vi "Primary Velocity.vi"(0 "Primary Average Density":dbl, 1 "Pipe X-SectionArea":dbl, 5 "Primary Hot Density":dbl, 7 "Primary Cold Density":dbl, 9 "Pri Mass Flow":dbl, 12 "RX X-Section":dbl, 13 "Numeric":dbl) -> (2 "Cold Leg Velocity (m/s)":dbl, 3 "Hot Leg Velocity (m/s)":dbl, 4 "MHX Velocity (m/s)":dbl, 6 "Velocity (m/s) 2":dbl, 8 "Velocity (m/s) 4":dbl, 10 "Velocity (m/s) 3":dbl, 14 "RX Velocity (m/s)":dbl, 15 "Velocity (m/s)":dbl)   [LabVIEW 2019]
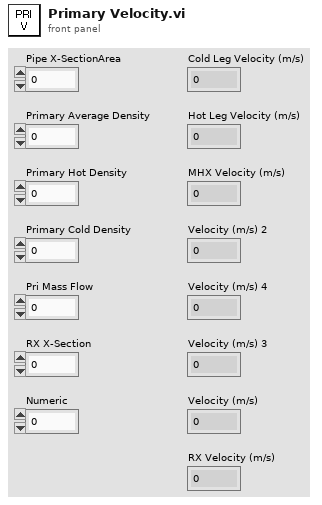
[diagram p1: front panel]
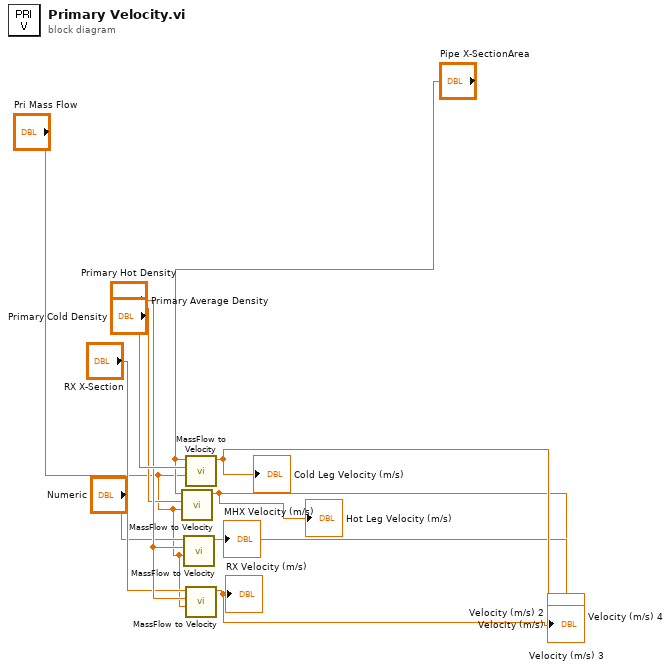
[diagram p0: block diagram]
diagram:
  n1 = call "MassFlow to Velocity.vi"("Mass Flow (kg/s)"="Pri Mass Flow", "Density (kg/m^3)"="Primary Hot Density", "Area (m^2)"="Pipe X-SectionArea") -> ("Velocity (m/s)"=→"Hot Leg Velocity (m/s)" →"Velocity (m/s) 4":dbl)  [unwired: 8 in]
  n2 = call "MassFlow to Velocity.vi"("Mass Flow (kg/s)"="Pri Mass Flow", "Density (kg/m^3)"="Primary Average Density", "Area (m^2)"="Numeric") -> ("Velocity (m/s)"=→"MHX Velocity (m/s)" →"Velocity (m/s) 3":dbl)  [unwired: 8 in]
  n3 = call "MassFlow to Velocity.vi"("Mass Flow (kg/s)"="Pri Mass Flow", "Density (kg/m^3)"="Primary Cold Density", "Area (m^2)"="Pipe X-SectionArea") -> ("Velocity (m/s)"=→"Cold Leg Velocity (m/s)" →"Velocity (m/s) 2":dbl)  [unwired: 8 in]
  n4 = call "MassFlow to Velocity.vi"("Mass Flow (kg/s)"="Pri Mass Flow", "Density (kg/m^3)"="Primary Average Density", "Area (m^2)"="RX X-Section") -> ("Velocity (m/s)"=→"RX Velocity (m/s)" →"Velocity (m/s)":dbl)  [unwired: 8 in]
